vi "control daq.vi"(0 "Camera Device IN":T4, 1 "Image Device IN":cluster{"Image":T3, "errorImage":errorcluster}, 2 "DAQ Device IN":T1={"DAQ Fs (S/s)"=10000.0, "task"="", "error"={"status"=FALSE, "code"=0, "source"=""}, "Min Value"=-10.0, "Max Value"=10.0}, 3 "Time Control Parameters":cluster{"# samples":u32, "tiempos (ms)":dbl}, 4 "Parametros Maximos":T5, 5 "detla Parametros":T5, 6 "Camara ON?":bool, 7 "Control Parameters":T2={"N Init Avg"=6, "N Avg Best"=3, "% Best to test"=0.95, "% Best to beat"=1.0}, 8 "Control?":bool=TRUE, 9 "Reset Control":bool, 10 "Ajuste?":bool=TRUE) -> (14 "Camara Device OUT":T4, 15 "Image Device OUT":cluster{"Image":T3, "errorImage":errorcluster}, 16 "DAQ Device OUT":T1={"DAQ Fs (S/s)"=0.0, "task"="", "error"={"status"=FALSE, "code"=0, "source"=""}, "Min Value"=-10.0, "Max Value"=10.0}, 17 "Contraste":dbl, 18 "Waveform":waveform(dbl), 19 "Señal de Control":dbl[](array[numeric]))   [LabVIEW 2010]
uses:
  <vilib>/vision/Image Controls.llb/IMAQ Image.ctl
  <vilib>/measure/NI_MABase.lvlib
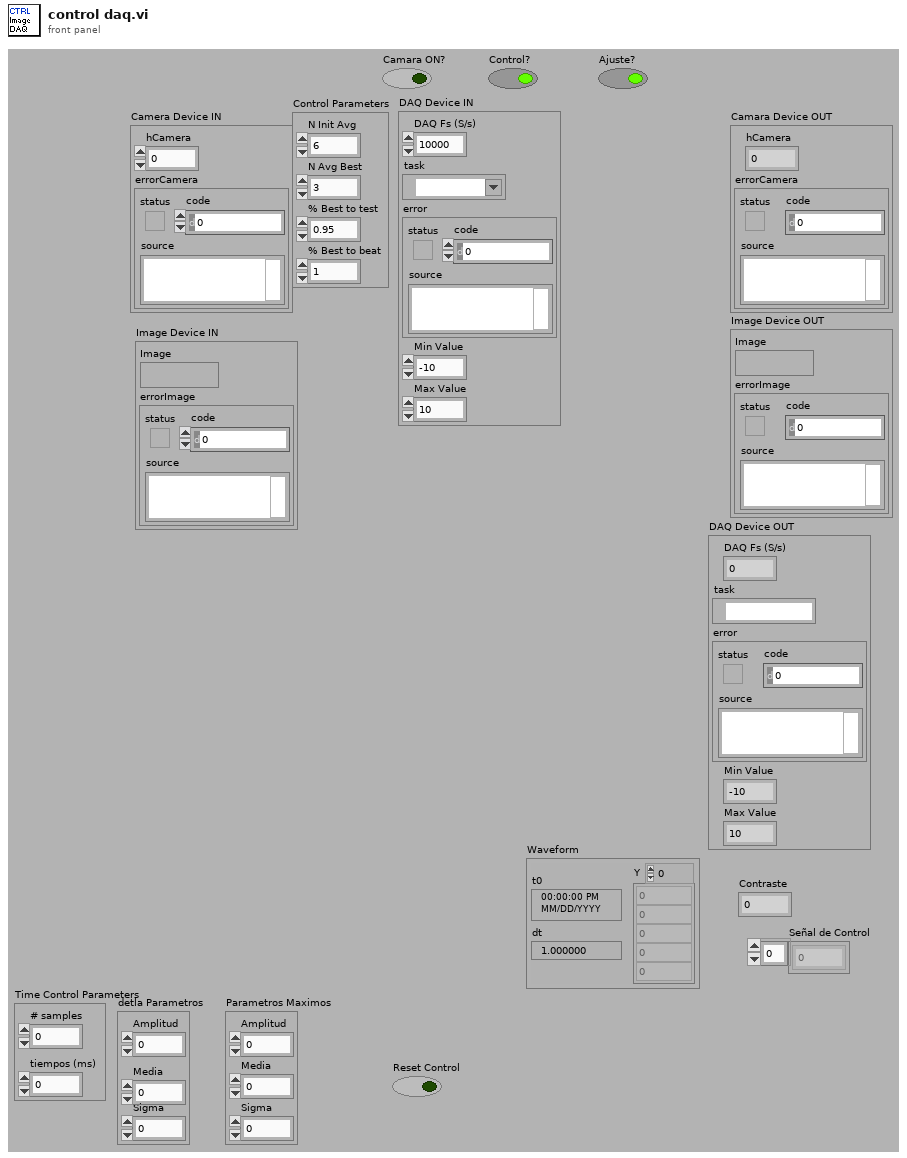
[diagram p1: front panel]
types:
  T1 = cluster{"DAQ Fs (S/s)":dbl, "task":refnum<k21>, "error":errorcluster, "Min Value":dbl, "Max Value":dbl}
  T2 = cluster{"N Init Avg":u32, "N Avg Best":u32, "% Best to test":dbl, "% Best to beat":dbl}
  T3 = typedef "IMAQ Image.ctl" = refnum<image>
  T4 = cluster{"hCamera":u32, "errorCamera":errorcluster}
  T5 = cluster{"Amplitud":dbl, "Media":dbl, "Sigma":dbl}
  T6 = cluster{"DAQ Limits":cluster{"max":dbl, "min":dbl}, "Control Limits":cluster{"max":dbl, "min":dbl}}
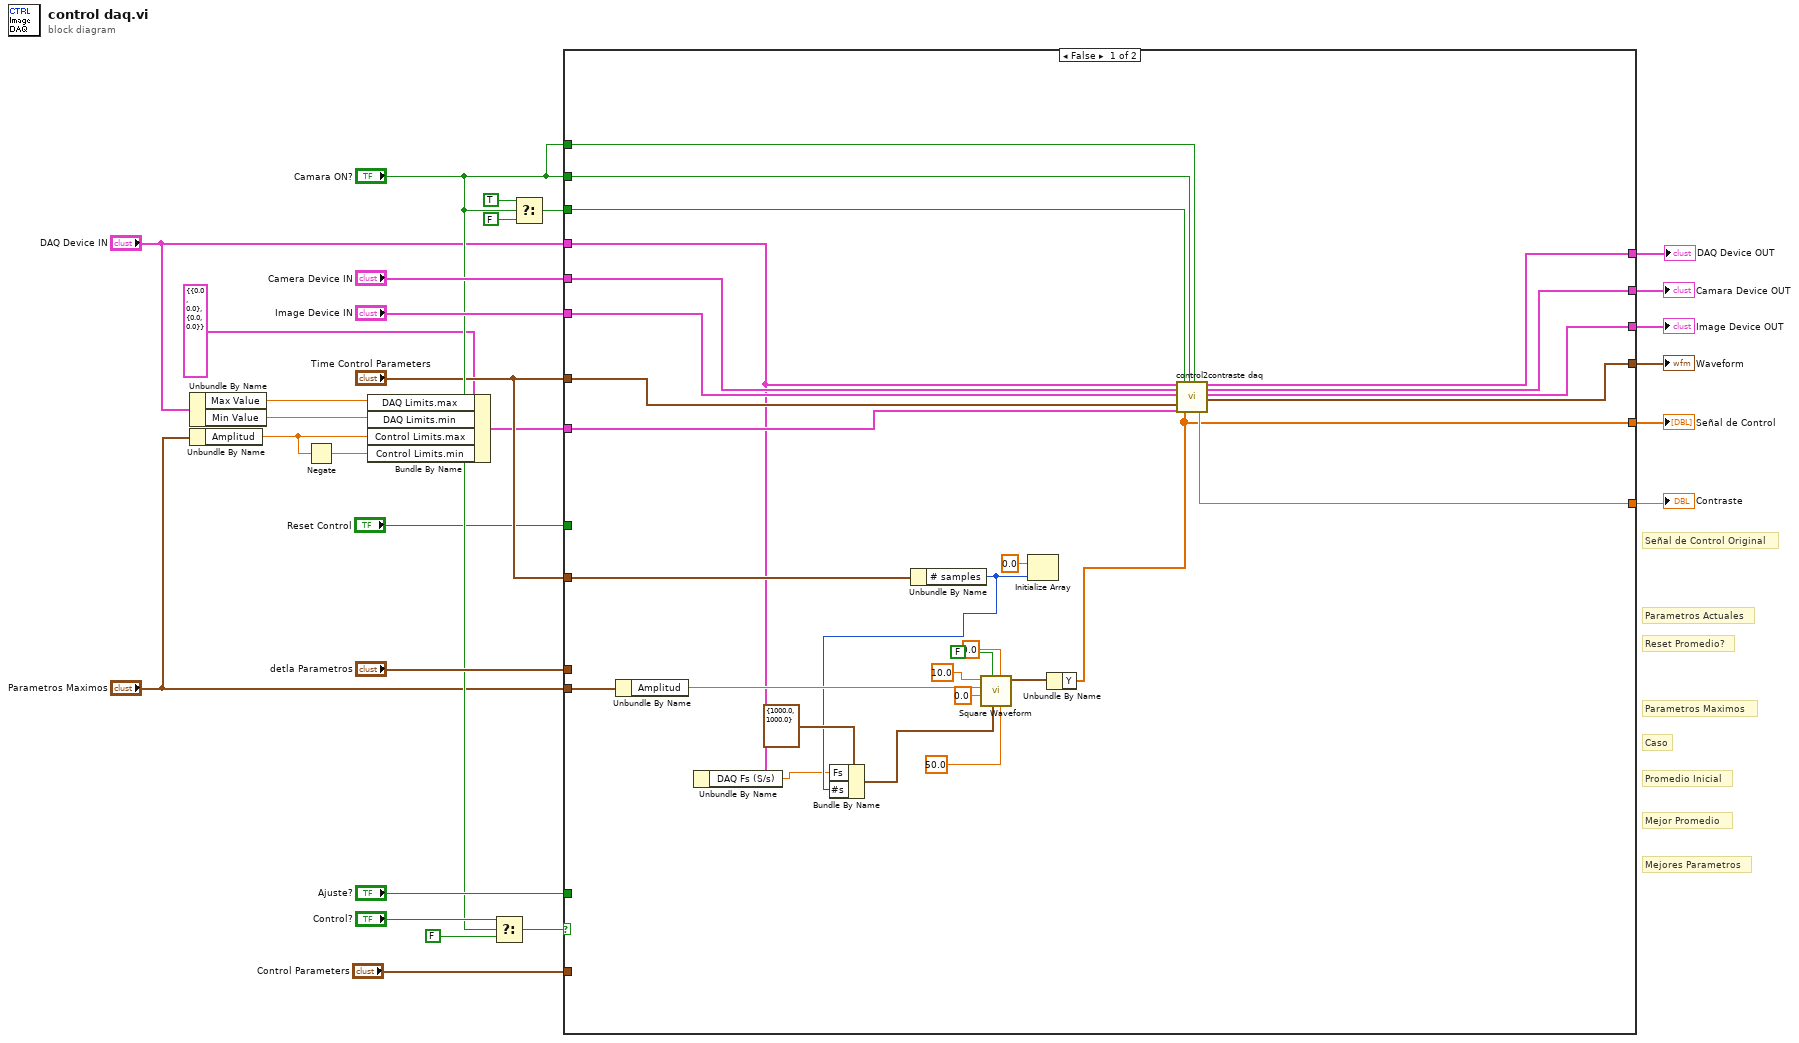
[diagram p0: block diagram]
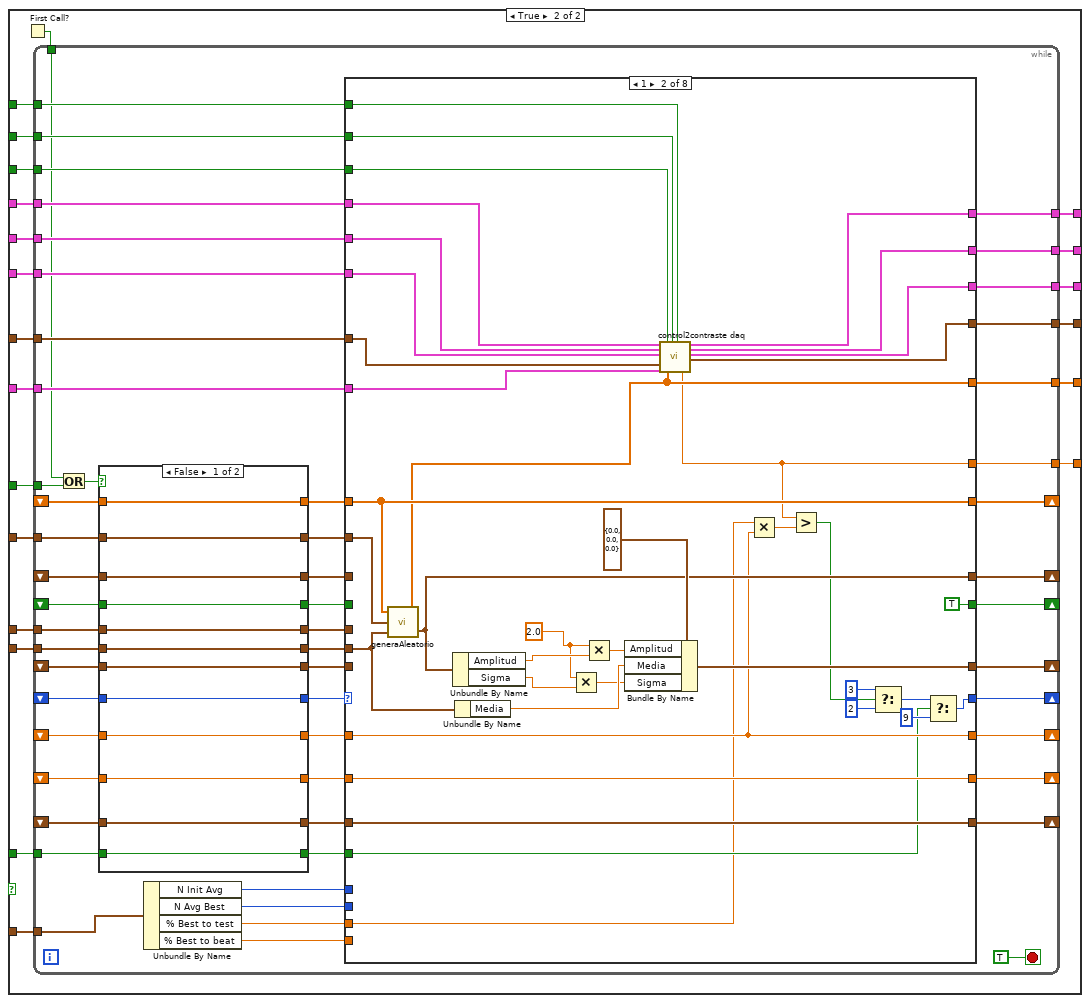
[diagram p2: hidden frame]
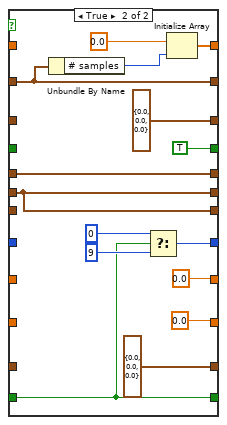
[diagram p3: hidden frame]
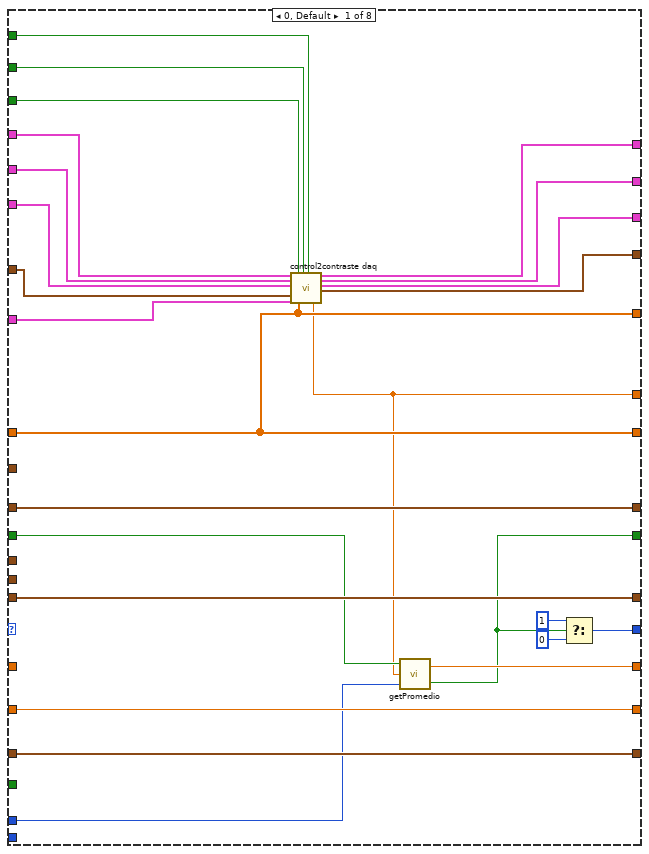
[diagram p4: hidden frame]
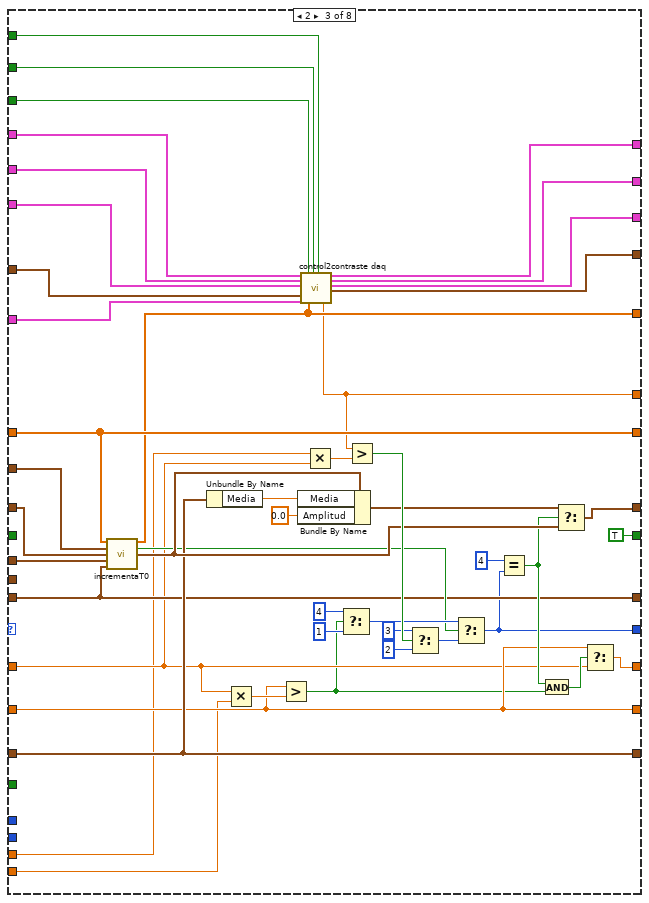
[diagram p5: hidden frame]
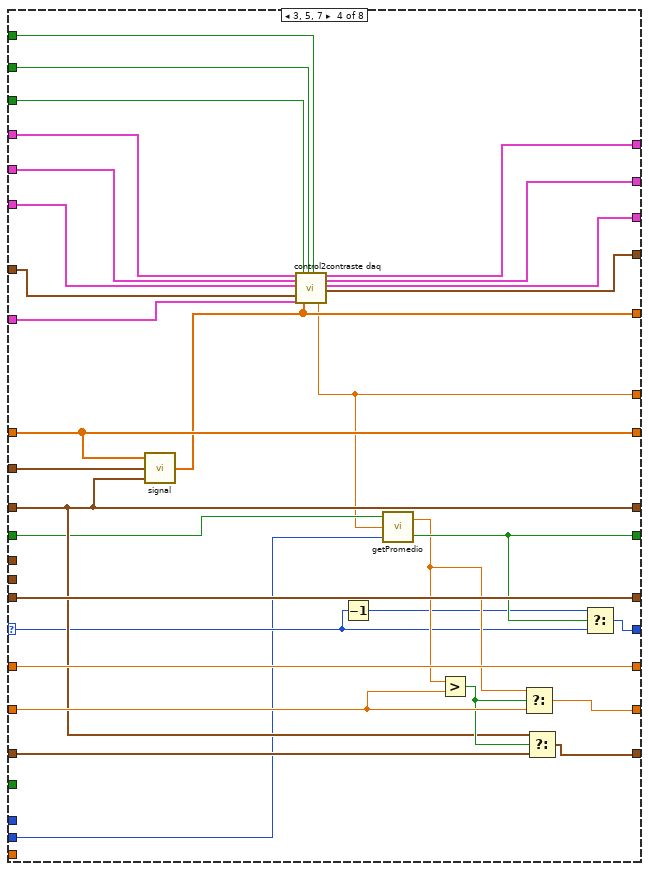
[diagram p6: hidden frame]
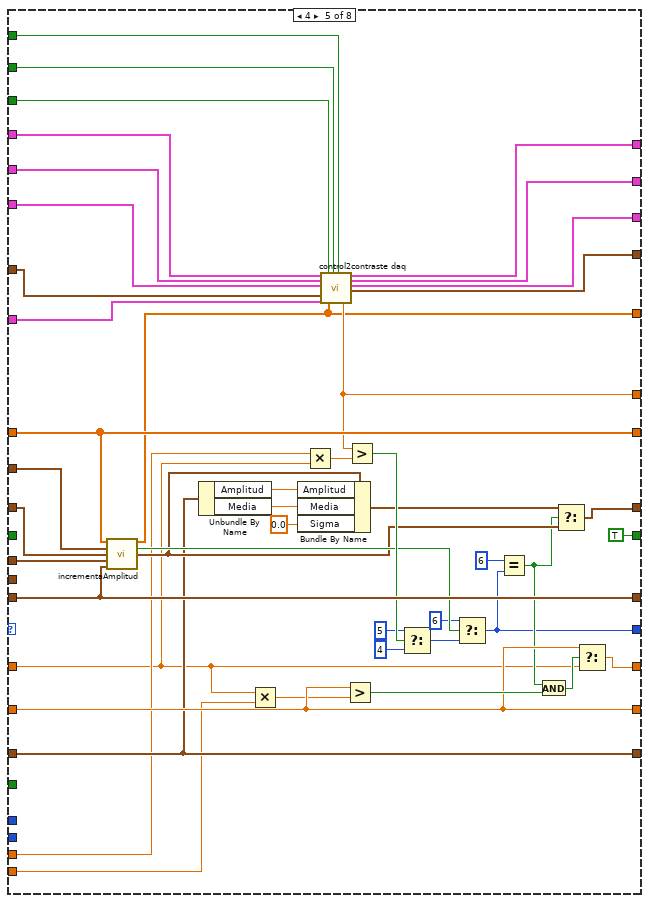
[diagram p7: hidden frame]
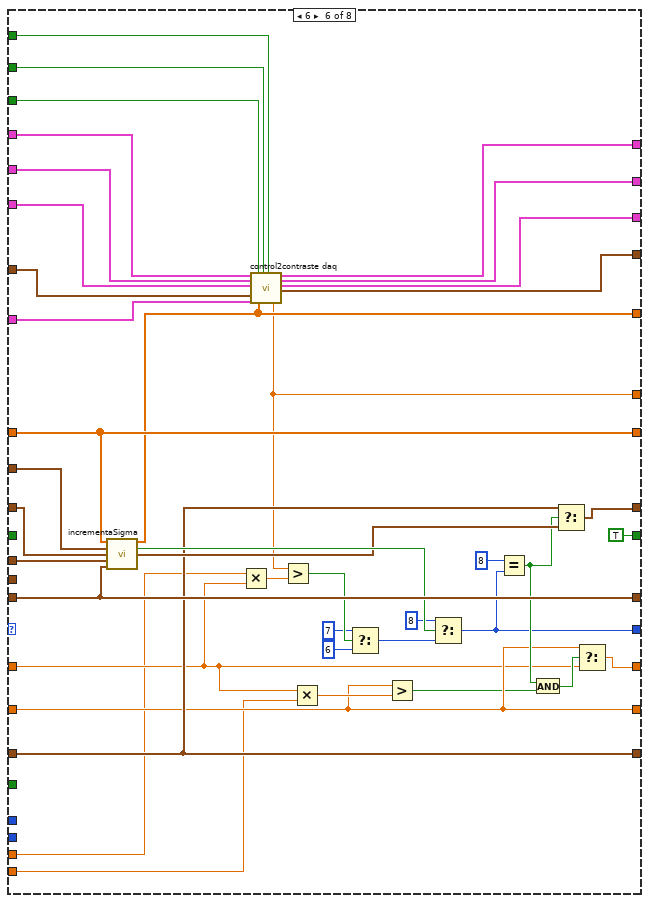
[diagram p8: hidden frame]
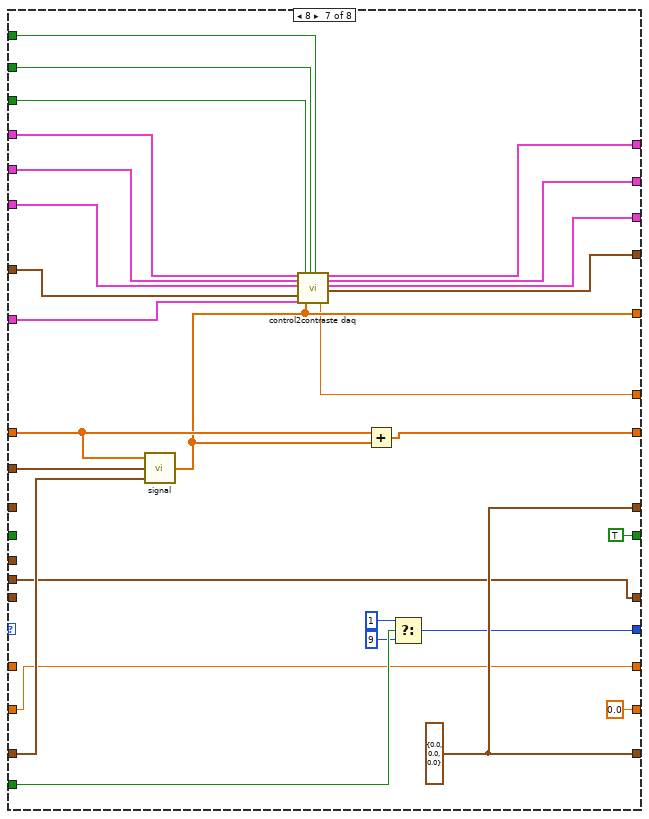
[diagram p9: hidden frame]
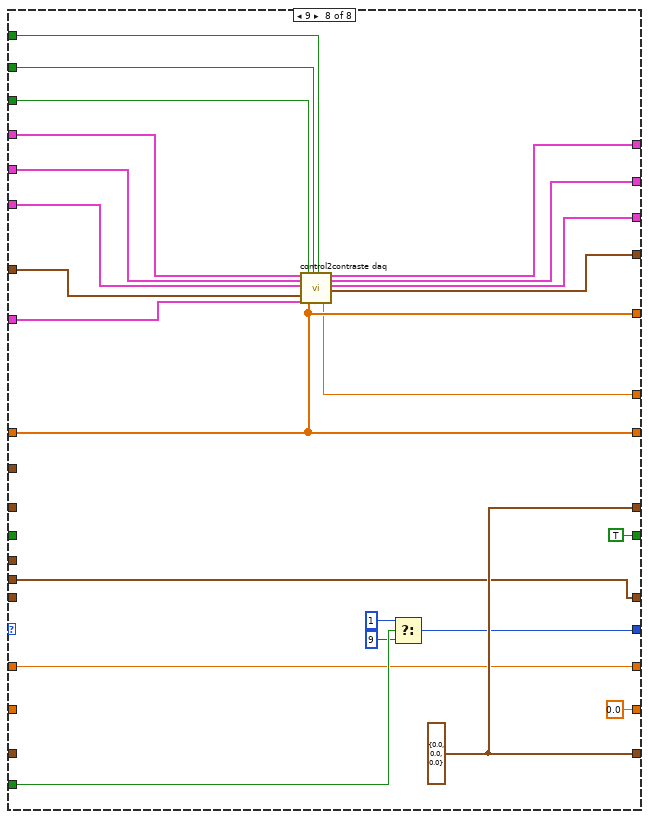
[diagram p10: hidden frame]
diagram:
  # "Reset Promedio?"
  # "Mejores Parametros"
  # "Mejor Promedio"
  # "Señal de Control Original"
  # "Parametros Actuales"
  # "Parametros Maximos"
  # "Caso"
  # "Promedio Inicial"
  n1 = Unbundle By Name("DAQ Device IN") -> ("Max Value"=w6:dbl, "Min Value"=w5:dbl)
  n2 = Unbundle By Name("Parametros Maximos") -> ("Amplitud"=w3:dbl)
  n3 = Negate(x=w3) -> (-x=w4:dbl)
  n4 = Bundle By Name(cluster=T6 {"DAQ Limits"={"max"=0.0, "min"=0.0}, "Control Limits"={"max"=0.0, "min"=0.0}} ("Limites"), "DAQ Limits.max"=w6, "DAQ Limits.min"=w5, "Control Limits.max"=w3, "Control Limits.min"=w4) -> (w7:T6)
  n5 = Select(t="Control?", s="Camara ON?", f=FALSE) -> (s? t:f=w16:bool)
  n6 = Select(t=TRUE, s="Camara ON?", f=FALSE) -> (s? t:f=w19:bool)
  n7 = case shown="False" w16 {
    tunnel: "Time Control Parameters" -> [w55 w77]
    tunnel: "detla Parametros" -> [_ w76]
    tunnel: "Parametros Maximos" -> [w41 w75]
    tunnel: "Ajuste?" -> [_ w73]
    tunnel: [w34 w72] -> w26
    tunnel: [w54 w71] -> w25
    tunnel: w7 -> [w53 w70]
    tunnel: "Time Control Parameters" -> [w52 w69]
    tunnel: "Image Device IN" -> [w51 w68]
    tunnel: "Camera Device IN" -> [w50 w67]
    tunnel: "DAQ Device IN" -> [w30 w66]
    tunnel: w19 -> [w49 w65]
    tunnel: "Camara ON?" -> [w48 w64]
    tunnel: "Camara ON?" -> [w47 w63]
    tunnel: [w46 w62] -> w22
    tunnel: [w45 w61] -> w21
    tunnel: [w44 w60] -> w20
    tunnel: [w43 w59] -> w9
    tunnel: "Reset Control" -> [_ w58]
    tunnel: "Control Parameters" -> [_ w57]
    frame False {
      n8 = Unbundle By Name(w41) -> ("Amplitud"=w40:dbl)
      n9 = Unbundle By Name(w30) -> ("DAQ Fs (S/s)"=w29:dbl)
      n10 = Unbundle By Name(w55) -> ("# samples"=w31:u32)
      n11 = Bundle By Name(cluster=cluster{"Fs":dbl, "#s":dbl} {"Fs"=1000.0, "#s"=1000.0} ("sampling info"), "Fs"=w29, "#s"=w31) -> (w32:cluster{"Fs":dbl, "#s":dbl})
      n12 = call <vilib>:"Square Waveform.vi"("duty cycle (%)"=50.0, "offset"=0.0, "sampling info"=w32, "reset signal"=FALSE, "phase"=0.0, "amplitude"=w40, "frequency"=10.0) -> ("signal out"=w35:waveform(dbl))  [unwired: 3 in, 1 out]
      n13 = Initialize Array(0.0 ("element"), w31) -> ()  [unwired: 1 out]
      n14 = Unbundle By Name(w35) -> ("Y"=w34:dbl[])
      n15 = call "control2contraste daq.vi"("DAQ Device IN"=w30, "Camera Device IN"=w50, "Image Device IN"=w51, "Time Control Parameters"=w52, "Limites"=w53, "DAQ?"=w49, "ControlSignal"=w34, "Streeam?"=w48, "Mostrar?"=w47) -> ("Contraste"=w54:dbl, "DAQ Device OUT"=w43:T1, "Camara Device OUT"=w44:T4, "Image Device OUT"=w45:cluster{"Image":T3, "errorImage":errorcluster}, "Waveform"=w46:waveform(dbl))  [unwired: 6 in]
    }
    frame True {
      n16 = First Call?() -> (First Call?: T/F=w74:bool)
      n17 = while {
        shift-right: [w129] -> _
        shift-left: _ -> [w116]
        tunnel: w77 -> [w108]
        shift-right: [w132] -> _
        shift-left: _ -> [w124]
        shift-right: [w131] -> _
        shift-left: _ -> [w118]
        shift-right: [w130] -> _
        shift-left: _ -> [w122]
        shift-right: [w128] -> _
        shift-left: _ -> [w114]
        tunnel: w76 -> [w105]
        shift-right: [w127] -> _
        shift-left: _ -> [w112]
        shift-right: [w126] -> _
        shift-left: _ -> [w110]
        shift-right: [w125] -> _
        shift-left: _ -> [w120]
        tunnel: w73 -> [w107]
        tunnel: w75 -> [w106]
        tunnel: w74 -> [w85]
        tunnel: [w100] -> w72
        tunnel: [w99] -> w71
        tunnel: w70 -> [w98]
        tunnel: w69 -> [w97]
        tunnel: w68 -> [w96]
        tunnel: w67 -> [w95]
        tunnel: w66 -> [w94]
        tunnel: w65 -> [w93]
        tunnel: w64 -> [w92]
        tunnel: w63 -> [w91]
        tunnel: [w90] -> w62
        tunnel: [w89] -> w61
        tunnel: [w88] -> w60
        tunnel: [w87] -> w59
        tunnel: w58 -> [w83]
        tunnel: w57 -> [w82]
        stop <- TRUE stop-if-true
        n18 = Or(x=w85, y=w83) -> (x .or. y?=w84:bool)
        n19 = case shown="False" w84 {
          tunnel: w124 -> [w144 _]
          tunnel: [w144 w159] -> w123
          tunnel: [w143 T5 {"Amplitud"=0.0, "Media"=0.0, "Sigma"=0.0} ("Parametros Iniciales")] -> w121
          tunnel: w122 -> [w143 _]
          tunnel: w120 -> [w142 _]
          tunnel: [w142 TRUE] -> w119
          tunnel: w118 -> [w141 _]
          tunnel: [w141 w148] -> w117
          tunnel: w116 -> [w140 _]
          tunnel: [w140 w149] -> w115
          tunnel: w114 -> [w139 _]
          tunnel: [w139 0.0 ("Contraste Promedio")] -> w113
          tunnel: w112 -> [w138 _]
          tunnel: [w138 0.0 ("Contraste Promedio")] -> w111
          tunnel: w110 -> [w137 _]
          tunnel: [w137 T5 {"Amplitud"=0.0, "Media"=0.0, "Sigma"=0.0} ("Parametros Maximos")] -> w109
          tunnel: w108 -> [w136 w145]
          tunnel: w106 -> [w134 w148]
          tunnel: w107 -> [w133 w146]
          tunnel: [w134 w148] -> w104
          tunnel: [w135 w147] -> w103
          tunnel: w105 -> [w135 w147]
          tunnel: [w133 w146] -> w102
          tunnel: [w136 w145] -> w101
          frame False {
          }
          frame True {
            n20 = Unbundle By Name(w145) -> ("# samples"=w157:u32)
            n21 = Select(t=u32 0, s=w146, f=u32 9) -> (s? t:f=w149:u32)
            n22 = Initialize Array(0.0 ("element"), w157) -> (w159:dbl[])
          }
        }
        n23 = Unbundle By Name(w82) -> ("N Init Avg"=w81:u32, "N Avg Best"=w80:u32, "% Best to test"=w79:dbl, "% Best to beat"=w78:dbl)
        n24 = case shown="1" w115 {
          selector: w115 -> [_ _ _ w285 _ _ _ _]
          tunnel: w123 -> [w174 w222 w266 w299 w342 w383 w405 w427]
          tunnel: w101 -> [_ w223 w269 w300 w345 w386 w413 _]
          tunnel: w117 -> [w177 _ w248 w291 w341 w382 _ _]
          tunnel: [w174 w222 w266 w299 w342 w383 w404 w427] -> w132
          tunnel: [w177 w221 w248 w291 w341 w382 w401 w429] -> w131
          tunnel: [w178 w219 w256 w290 w331 w374 w410 w435] -> w130
          tunnel: [w184 w186 w231 w298 w308 w352 w402 w430] -> w129
          tunnel: [w179 w209 w260 w297 w336 w378 w403 w428] -> w128
          tunnel: w113 -> [_ w209 w226 w297 w301 w348 _ w428]
          tunnel: [w173 w187 w246 w283 w322 w368 w399 w426] -> w99
          tunnel: [w174 w203 w247 w284 w321 w369 w400 w427] -> w100
          tunnel: w121 -> [w178 _ w268 w290 w344 w385 _ _]
          tunnel: w103 -> [_ _ w267 _ w343 w384 _ _]
          tunnel: [w180 w212 w228 w296 w334 w350 0.0 ("Contraste Promedio") 0.0 ("Contraste Promedio")] -> w127
          tunnel: [w181 w211 w253 w294 w328 w370 w410 w435] -> w126
          tunnel: w109 -> [w181 w211 w253 w292 w328 w370 w412 _]
          tunnel: w111 -> [w180 w212 w228 w295 w334 w350 w403 _]
          tunnel: w119 -> [w175 _ _ w289 _ _ _ _]
          tunnel: [w176 TRUE ("Llego a N?") TRUE ("Llego a N?") w288 TRUE ("Llego a N?") TRUE ("Llego a N?") TRUE ("Llego a N?") TRUE ("Llego a N?")] -> w125
          tunnel: w102 -> [_ w188 _ _ _ _ w408 w433]
          tunnel: w104 -> [_ w204 _ _ _ _ w401 w429]
          tunnel: w98 -> [w172 w202 w245 w282 w305 w367 w398 w425]
          tunnel: w97 -> [w171 w201 w244 w281 w306 w363 w397 w424]
          tunnel: w96 -> [w170 w200 w243 w280 w320 w362 w396 w423]
          tunnel: w95 -> [w169 w199 w242 w279 w319 w361 w395 w422]
          tunnel: w94 -> [w168 w191 w241 w278 w307 w360 w394 w421]
          tunnel: w93 -> [w167 w198 w240 w277 w318 w364 w393 w420]
          tunnel: w92 -> [w166 w197 w239 w276 w317 w365 w392 w419]
          tunnel: w91 -> [w165 w196 w238 w275 w316 w366 w391 w418]
          tunnel: [w164 w195 w237 w274 w315 w359 w390 w417] -> w90
          tunnel: [w163 w193 w236 w273 w314 w358 w389 w416] -> w89
          tunnel: [w162 w194 w235 w272 w313 w357 w388 w415] -> w88
          tunnel: [w161 w192 w234 w271 w312 w356 w387 w414] -> w87
          tunnel: w81 -> [w160 _ _ _ _ _ _ _]
          tunnel: w80 -> [_ _ _ w270 _ _ _ _]
          tunnel: w79 -> [_ w185 w224 _ w304 w347 _ _]
          tunnel: w78 -> [_ _ w227 _ w303 w349 _ _]
          frame 0, Default {
            n25 = call "control2contraste daq.vi"("DAQ Device IN"=w168, "Camera Device IN"=w169, "Image Device IN"=w170, "Time Control Parameters"=w171, "Limites"=w172, "DAQ?"=w167, "ControlSignal"=w174, "Streeam?"=w166, "Mostrar?"=w165) -> ("Contraste"=w173:dbl, "DAQ Device OUT"=w161:T1, "Camara Device OUT"=w162:T4, "Image Device OUT"=w163:cluster{"Image":T3, "errorImage":errorcluster}, "Waveform"=w164:waveform(dbl))  [unwired: 6 in]
            n26 = call "getPromedio.vi"("N"=w160, "Contraste"=w173, "Reset"=w175) -> ("Llego a N?"=w176:bool, "Contraste Promedio"=w179:dbl)
            n27 = Select(t=u32 1, s=w176, f=u32 0) -> (s? t:f=w184:u32)
          }
          frame 1 {
            w214 = 2.0 ("x")
            n28 = call "generaAleatorio.vi"("Parametros Maximos"=w204, "Sound Parameters"=w223, "Señal de Control IN"=w222) -> ("Parametros Iniciales"=w219:T5, "Out"=w203:dbl[])
            n29 = Unbundle By Name(w219) -> ("Amplitud"=w218:dbl, "Sigma"=w215:dbl)
            n30 = Unbundle By Name(w204) -> ("Media"=w216:dbl)
            n31 = Multiply(x=w214, y=w215) -> (x*y=w213:dbl)
            n32 = Multiply(x=w214, y=w218) -> (x*y=w217:dbl)
            n33 = Bundle By Name(cluster=T5 {"Amplitud"=0.0, "Media"=0.0, "Sigma"=0.0} ("Parametros Iniciales"), "Amplitud"=w217, "Media"=w216, "Sigma"=w213) -> (w221:T5)
            n34 = call "control2contraste daq.vi"("DAQ Device IN"=w191, "Camera Device IN"=w199, "Image Device IN"=w200, "Time Control Parameters"=w201, "Limites"=w202, "DAQ?"=w198, "ControlSignal"=w203, "Streeam?"=w197, "Mostrar?"=w196) -> ("Contraste"=w187:dbl, "DAQ Device OUT"=w192:T1, "Camara Device OUT"=w194:T4, "Image Device OUT"=w193:cluster{"Image":T3, "errorImage":errorcluster}, "Waveform"=w195:waveform(dbl))  [unwired: 6 in]
            n35 = Multiply(x=w185, y=w209) -> (x*y=w210:dbl)
            n36 = Greater?(x=w187, y=w210) -> (0:w208:bool)
            n37 = Select(t=u32 3, s=w208, f=u32 2) -> (s? t:f=w189:u32)
            n38 = Select(t=w189, s=w188, f=u32 9) -> (s? t:f=w186:u32)
          }
          frame 2 {
            n39 = call "incrementaT0.vi"("Señal de Control IN"=w266, "Sound Parameters"=w269, "Parametros Actuales IN"=w268, "detla Parametros"=w267, "Parametros Maximos"=w248) -> ("Out"=w247:dbl[], "Tope?"=w250:bool, "Parametros Actuales OUT"=w254:T5)  [unwired: 8 in]
            n40 = Unbundle By Name(w253) -> ("Media"=w252:dbl)
            n41 = Multiply(x=w226, y=w227) -> (x*y=w229:dbl)
            n42 = Greater?(x=w228, y=w229) -> (0:w225:bool)
            n43 = Bundle By Name(cluster=w254, "Media"=w252, "Amplitud"=0.0) -> (w255:T5)
            n44 = call "control2contraste daq.vi"("DAQ Device IN"=w241, "Camera Device IN"=w242, "Image Device IN"=w243, "Time Control Parameters"=w244, "Limites"=w245, "DAQ?"=w240, "ControlSignal"=w247, "Streeam?"=w239, "Mostrar?"=w238) -> ("Contraste"=w246:dbl, "DAQ Device OUT"=w234:T1, "Camara Device OUT"=w235:T4, "Image Device OUT"=w236:cluster{"Image":T3, "errorImage":errorcluster}, "Waveform"=w237:waveform(dbl))  [unwired: 6 in]
            n45 = Multiply(x=w224, y=w226) -> (x*y=w265:dbl)
            n46 = Select(t=u32 4, s=w225, f=u32 1) -> (s? t:f=w261:u32)
            n47 = Greater?(x=w246, y=w265) -> (0:w264:bool)
            n48 = Select(t=u32 3, s=w264, f=u32 2) -> (s? t:f=w230:u32)
            n49 = Select(t=w261, s=w250, f=w230) -> (s? t:f=w231:u32)
            n50 = Equal?(x=u32 4, y=w231) -> (x = y?=w249:bool)
            n51 = And(x=w249, y=w225) -> (x .and. y?=w259:bool)
            n52 = Select(t=w255, s=w249, f=w254) -> (s? t:f=w256:T5)
            n53 = Select(t=w228, s=w259, f=w226) -> (s? t:f=w260:dbl)
          }
          frame 3, 5, 7 {
            n54 = call "signal.vi"("Parametros Actuales IN"=w290, "Sound Parameters"=w300, "Señal de Control IN"=w299) -> ("Out"=w284:dbl[])
            n55 = call "control2contraste daq.vi"("DAQ Device IN"=w278, "Camera Device IN"=w279, "Image Device IN"=w280, "Time Control Parameters"=w281, "Limites"=w282, "DAQ?"=w277, "ControlSignal"=w284, "Streeam?"=w276, "Mostrar?"=w275) -> ("Contraste"=w283:dbl, "DAQ Device OUT"=w271:T1, "Camara Device OUT"=w272:T4, "Image Device OUT"=w273:cluster{"Image":T3, "errorImage":errorcluster}, "Waveform"=w274:waveform(dbl))  [unwired: 6 in]
            n56 = Decrement(x=w285) -> (x-1=w286:u32)
            n57 = call "getPromedio.vi"("N"=w270, "Contraste"=w283, "Reset"=w289) -> ("Llego a N?"=w288:bool, "Contraste Promedio"=w287:dbl)
            n58 = Greater?(x=w287, y=w295) -> (0:w293:bool)
            n59 = Select(t=w287, s=w293, f=w295) -> (s? t:f=w296:dbl)
            n60 = Select(t=w290, s=w293, f=w292) -> (s? t:f=w294:T5)
            n61 = Select(t=w286, s=w288, f=w285) -> (s? t:f=w298:u32)
          }
          frame 4 {
            n62 = call "incrementaAmplitud.vi"("Señal de Control IN"=w342, "Sound Parameters"=w345, "Parametros Actuales IN"=w344, "detla Parametros"=w343, "Parametros Maximos"=w341) -> ("Out"=w321:dbl[], "Tope?"=w338:bool, "Parametros Actuales OUT"=w329:T5)  [unwired: 8 in]
            n63 = Unbundle By Name(w328) -> ("Amplitud"=w327:dbl, "Media"=w325:dbl)
            n64 = Multiply(x=w301, y=w303) -> (x*y=w302:dbl)
            n65 = Bundle By Name(cluster=w329, "Amplitud"=w327, "Media"=w325, "Sigma"=0.0 ("Amplitud")) -> (w330:T5)
            n66 = Multiply(x=w304, y=w301) -> (x*y=w340:dbl)
            n67 = call "control2contraste daq.vi"("DAQ Device IN"=w307, "Camera Device IN"=w319, "Image Device IN"=w320, "Time Control Parameters"=w306, "Limites"=w305, "DAQ?"=w318, "ControlSignal"=w321, "Streeam?"=w317, "Mostrar?"=w316) -> ("Contraste"=w322:dbl, "DAQ Device OUT"=w312:T1, "Camara Device OUT"=w313:T4, "Image Device OUT"=w314:cluster{"Image":T3, "errorImage":errorcluster}, "Waveform"=w315:waveform(dbl))  [unwired: 6 in]
            n68 = Greater?(x=w334, y=w302) -> (0:w337:bool)
            n69 = Greater?(x=w322, y=w340) -> (0:w339:bool)
            n70 = Select(t=u32 5, s=w339, f=u32 4) -> (s? t:f=w309:u32)
            n71 = Select(t=u32 6, s=w338, f=w309) -> (s? t:f=w308:u32)
            n72 = Equal?(x=u32 6, y=w308) -> (x = y?=w323:bool)
            n73 = And(x=w323, y=w337) -> (x .and. y?=w335:bool)
            n74 = Select(t=w330, s=w323, f=w329) -> (s? t:f=w331:T5)
            n75 = Select(t=w334, s=w335, f=w301) -> (s? t:f=w336:dbl)
          }
          frame 6 {
            n76 = call "incrementaSigma.vi"("Señal de Control IN"=w383, "Sound Parameters"=w386, "Parametros Actuales IN"=w385, "detla Parametros"=w384, "Parametros Maximos"=w382) -> ("Out"=w369:dbl[], "Tope?"=w379:bool, "Parametros Actuales OUT"=w373:T5)  [unwired: 8 in]
            n77 = Multiply(x=w347, y=w348) -> (x*y=w381:dbl)
            n78 = call "control2contraste daq.vi"("DAQ Device IN"=w360, "Camera Device IN"=w361, "Image Device IN"=w362, "Time Control Parameters"=w363, "Limites"=w367, "DAQ?"=w364, "ControlSignal"=w369, "Streeam?"=w365, "Mostrar?"=w366) -> ("Contraste"=w368:dbl, "DAQ Device OUT"=w356:T1, "Camara Device OUT"=w357:T4, "Image Device OUT"=w358:cluster{"Image":T3, "errorImage":errorcluster}, "Waveform"=w359:waveform(dbl))  [unwired: 6 in]
            n79 = Greater?(x=w368, y=w381) -> (0:w380:bool)
            n80 = Multiply(x=w348, y=w349) -> (x*y=w351:dbl)
            n81 = Select(t=u32 7, s=w380, f=u32 6) -> (s? t:f=w353:u32)
            n82 = Greater?(x=w350, y=w351) -> (0:w346:bool)
            n83 = Select(t=u32 8, s=w379, f=w353) -> (s? t:f=w352:u32)
            n84 = Equal?(x=u32 8, y=w352) -> (x = y?=w371:bool)
            n85 = And(x=w371, y=w346) -> (x .and. y?=w377:bool)
            n86 = Select(t=w370, s=w371, f=w373) -> (s? t:f=w374:T5)
            n87 = Select(t=w350, s=w377, f=w348) -> (s? t:f=w378:dbl)
          }
          frame 8 {
            w410 = T5 {"Amplitud"=0.0, "Media"=0.0, "Sigma"=0.0} ("Parametros Maximos")
            n88 = call "signal.vi"("Parametros Actuales IN"=w412, "Sound Parameters"=w413, "Señal de Control IN"=w405) -> ("Out"=w400:dbl[])
            n89 = call "control2contraste daq.vi"("DAQ Device IN"=w394, "Camera Device IN"=w395, "Image Device IN"=w396, "Time Control Parameters"=w397, "Limites"=w398, "DAQ?"=w393, "ControlSignal"=w400, "Streeam?"=w392, "Mostrar?"=w391) -> ("Contraste"=w399:dbl, "DAQ Device OUT"=w387:T1, "Camara Device OUT"=w388:T4, "Image Device OUT"=w389:cluster{"Image":T3, "errorImage":errorcluster}, "Waveform"=w390:waveform(dbl))  [unwired: 6 in]
            n90 = Add(x=w405, y=w400) -> (x+y=w404:dbl[])
            n91 = Select(t=u32 1, s=w408, f=u32 9) -> (s? t:f=w402:u32)
          }
          frame 9 {
            w435 = T5 {"Amplitud"=0.0, "Media"=0.0, "Sigma"=0.0} ("Parametros Maximos")
            n92 = call "control2contraste daq.vi"("DAQ Device IN"=w421, "Camera Device IN"=w422, "Image Device IN"=w423, "Time Control Parameters"=w424, "Limites"=w425, "DAQ?"=w420, "ControlSignal"=w427, "Streeam?"=w419, "Mostrar?"=w418) -> ("Contraste"=w426:dbl, "DAQ Device OUT"=w414:T1, "Camara Device OUT"=w415:T4, "Image Device OUT"=w416:cluster{"Image":T3, "errorImage":errorcluster}, "Waveform"=w417:waveform(dbl))  [unwired: 6 in]
            n93 = Select(t=u32 1, s=w433, f=u32 9) -> (s? t:f=w430:u32)
          }
        }
      }
    }
  }
  "Señal de Control" <- w26
  "Contraste" <- w25
  "Camara Device OUT" <- w20
  "Image Device OUT" <- w21
  "Waveform" <- w22
  "DAQ Device OUT" <- w9
